vi "ConfigFolder.vi"(11 "error in (no error)":errorcluster) -> (4 "dup path":path, 15 "error out":errorcluster)   [LabVIEW 2019]
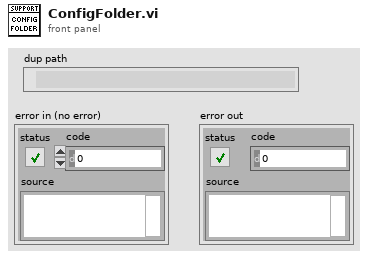
[diagram p1: front panel]
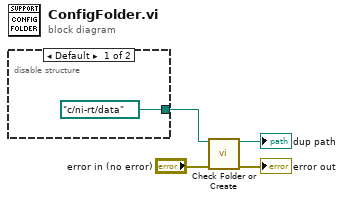
[diagram p0: block diagram]
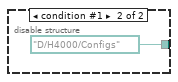
[diagram p2: hidden frame]
diagram:
  n1 = disable-structure shown="Default" {
    disable-tunnel: [path "c:/ni-rt/data" ("Config Dir") path "D:/H4000/Configs" ("Config Dir")] -> w4
    frame condition #0 (active) {
    }
    frame condition #1 {
    }
  }
  n2 = call "Check Folder or Create.vi"("path"=w4, "error in (no error)"="error in (no error)") -> ("dup path"=→"dup path":path, "error out"=→"error out":errorcluster)  [unwired: 12 in]
